vi "Word Report - Run Macro.vi"() -> ()   [LabVIEW 2023]
doc: "This example inserts a table into a new Word document, imports a Visual Basic module into the document, executes a macro contained in the module to process the table and removes the module from the document."
uses:
  <vilib>/Utility/NIReport.llb/Report Type.ctl
  <vilib>/Utility/NIReport.llb/NI_report.lvclass
  <vilib>/Utility/NIReport.llb/Word/NI_Word.lvclass
  <vilib>/Utility/NIReport.llb/NI_ReportGenerationCore.lvlib
panel:
  in  "Module Code":string="Sub ProcessTable()\n\nActiveDocument.Tables.Item(1).Borders.OutsideLineWidth = wdLineWidth300pt\n\nEnd Sub"
  # "Overview: This example imports a Visual Basic module into the document and executes a macro contained in the module in order to process a table.  Then it removes the module from the document.\nRequirements: Report Generation Toolkit, Microsoft Word\nInstructions:\nRun the VI.\n\nNote: \n1. Ensure you have enabled all macros in the Word Trust Center. To do this, go to File > Options > Trust Center > Trust Center Settings > Macro Settings and select Enable all macros. You should also select Trust access to the VBA project object model.\n2. Run the VI.\n3. (Optional) Restore your previous macro security settings in Microsoft Word."
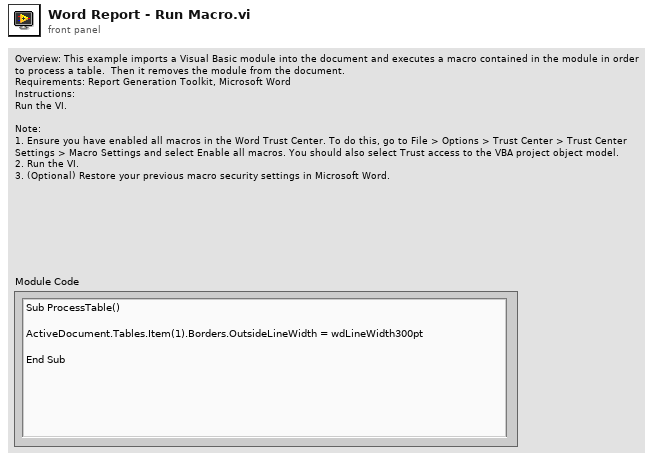
[diagram p1: front panel]
types:
  T1 = typedef "NI_ReportGenerationCore.lvlib/Report Type.ctl" = enum16{"HTML", "Word", "Excel"}
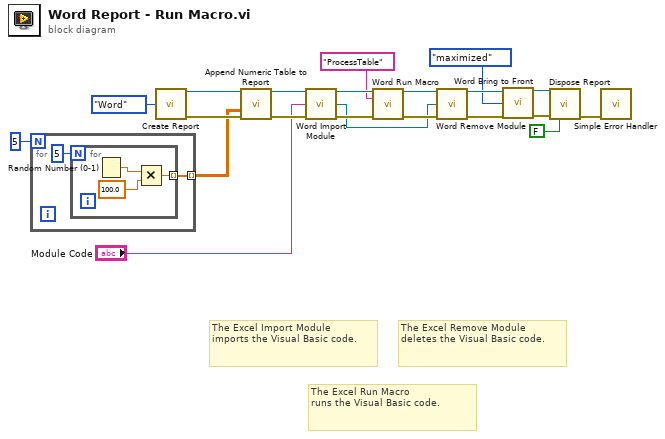
[diagram p0: block diagram]
diagram:
  # "The Excel Remove Module\ndeletes the Visual Basic code."
  # "The Excel Run Macro\nruns the Visual Basic code."
  # "The Excel Import Module\nimports the Visual Basic code."
  n1 = for {
    N: 5 -> [_]
    tunnel: [w22] -> w2 mode=indexing
    n2 = for {
      N: 5 ("dimension size") -> [_]
      tunnel: [w24] -> w22 mode=indexing
      n3 = Random Number (0-1)() -> (number: 0 to 1=w26:dbl)
      n4 = Multiply(x=w26, y=100.0) -> (x*y=w24:dbl)
    }
  }
  n5 = call <vilib>:"Create Report.vi"("report type"=Report_Type."Word" ("Report Type")) -> ("report out"=w15:refnum<class "NI_report.lvclass">, "error out"=w16:errorcluster)  [unwired: 13 in]
  n6 = call-dynamic "Append Numeric Table to Report.vi"("report in"=w15, "numerical data"=w2, "error in (no error)"=w16) -> ("report out"=w18:refnum<class "NI_report.lvclass">, "error out"=w19:errorcluster)  [unwired: 9 in, 2 out]
  n7 = call <vilib>:"Word Import Module.vi"("report in"=w18, "module code (\"\")"="Module Code", "error in (no error)"=w19) -> ("report out"=w20:refnum<class "NI_report.lvclass">, "module reference"=w12:refnum<k7>, "error out"=w21:errorcluster)  [unwired: 10 in]
  n8 = call <vilib>:"Word Run Macro.vi"("report in"=w20, "macro name"="ProcessTable" ("Macro"), "error in (no error)"=w21) -> ("report out"=w13:refnum<class "NI_report.lvclass">, "error out"=w14:errorcluster)  [unwired: 10 in, 1 out]
  n9 = call <vilib>:"Word Remove Module.vi"("report in"=w13, "module reference"=w12, "error in (no error)"=w14) -> ("report out"=w10:refnum<class "NI_report.lvclass">, "error out"=w11:errorcluster)  [unwired: 11 in]
  n10 = call <vilib>:"Word Bring to Front.vi"("report in"=w10, "window state (maximized)"=enum16{"maximized", "minimized", "normal"}."maximized", "error in (no error)"=w11) -> ("report out"=w8:refnum<class "NI_report.lvclass">, "error out"=w7:errorcluster)  [unwired: 11 in]
  n11 = call-dynamic "Dispose Report.vi"("report in"=w8, "error in (no error)"=w7, "close report? (T)"=FALSE ("Close Report? (T)")) -> ("error out"=w6:errorcluster)  [unwired: 12 in]
  n12 = call <vilib>:"Simple Error Handler.vi"("error in (no error)"=w6) -> ()  [unwired: 4 in, 5 out]
